vi "IT6700H Output DC Volts.vi"() -> ()   [LabVIEW 2015]
doc: "This example shows how to configure the instrument's output voltage level, over current protection, and over voltage protection. The actual voltage level and actual current level are returned as well as whether over voltage protection (OVP) or over current protection (OCP) has been tripped."
uses:
  <instrlib>/IT6700H/IT6700H.lvlib
panel:
  in  "OCP Level(A)":dbl min=0.0 format="%.2g"
  in  "OCP State":bool
  in  "OVP Level(V)":dbl min=0.0 format="%.2g"
  in  "OVP State":bool
  in  "Serial Configuration":T1={"Baud Rate"=9600, "Parity"=0, "Data Bits"=8, "Stop Bits"=10, "Flow Control"=0} {"Flow Control" items=["None", "XON/XOFF", "RTS/CTS", "XON/XOFF & RTS/CTS", "DTR/DSR", "XON/XOFF & DTR/DSR"]; "Stop Bits" items=["1.0"=10, "1.5"=15, "2.0"=20]; "Data Bits" items=["7"=7, "8"=8]; "Parity" items=["None", "Odd", "Even", "Mark", "Space"]; "Baud Rate" items=["300"=300, "600"=600, "1200"=1200, "2400"=2400, "4800"=4800, "9600"=9600, "19200"=19200]}
  in  "Stop Output":bool
  in  "Voltage(V)":dbl=1.0 min=0.0 format="%.2f"
  out "Read Current(A)":dbl format="%.3f"
  out "Read Voltage(V)":dbl format="%.3f"
  in  "Current(A)":dbl=1.0 min=0.0 format="%.2f"
  in  "VISA resource name":refnum<visa-resource-name>
  # "Source Output"
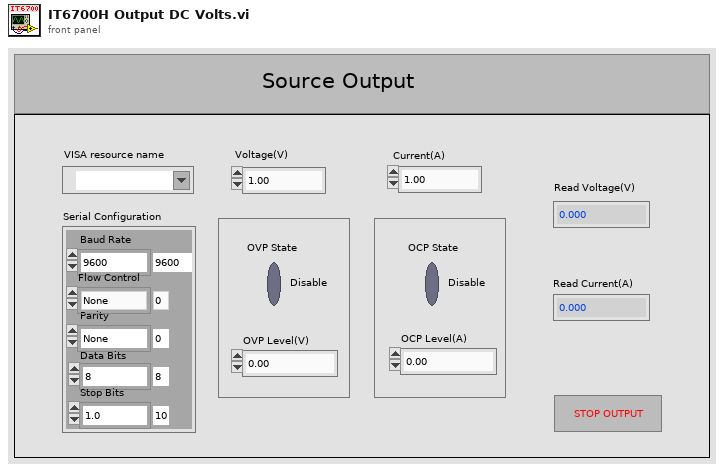
[diagram p1: front panel]
types:
  T1 = cluster{"Baud Rate":u32, "Parity":u16, "Data Bits":u16, "Stop Bits":u16, "Flow Control":u16}
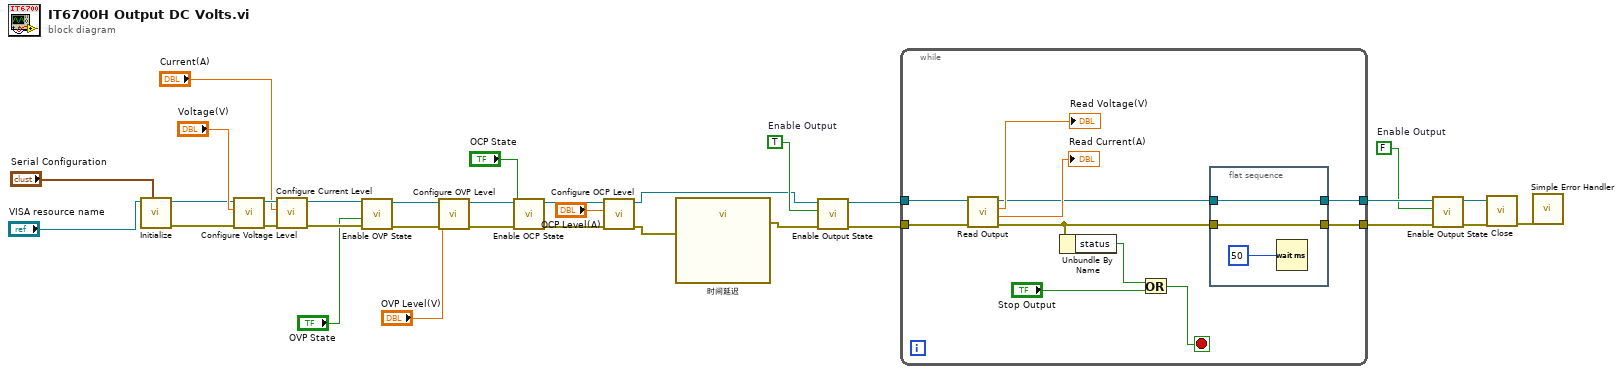
[diagram p0: block diagram]
diagram:
  w18 = FALSE  # Enable Output
  w23 = TRUE  # Enable Output
  n1 = call <instrlib>:"Initialize.vi"("Serial Configuration"="Serial Configuration", "VISA resource name"="VISA resource name") -> ("error out"=w16:errorcluster, "VISA resource name out"=w17:refnum<visa-resource-name>)  [unwired: 8 in]
  n2 = call <instrlib>:"Configure Voltage Level.vi"("error in"=w16, "Voltage(V)"="Voltage(V)", "VISA resource name"=w17) -> ("error out"=w29:errorcluster, "VISA resource name out"=w28:refnum<visa-resource-name>)  [unwired: 7 in]
  n3 = call <instrlib>:"Configure Current Level.vi"("error in"=w29, "Current(A)"="Current(A)", "VISA resource name"=w28) -> ("error out"=w14:errorcluster, "VISA resource name out"=w15:refnum<visa-resource-name>)  [unwired: 7 in]
  n4 = call <instrlib>:"Enable OVP State.vi"("error in"=w14, "State"="OVP State", "VISA resource name"=w15) -> ("error out"=w11:errorcluster, "VISA resource name out"=w12:refnum<visa-resource-name>)  [unwired: 7 in]
  n5 = call <instrlib>:"Configure OVP Level.vi"("error in"=w11, "Level(V)"="OVP Level(V)", "VISA resource name"=w12) -> ("error out"=w8:errorcluster, "VISA resource name out"=w9:refnum<visa-resource-name>)  [unwired: 7 in]
  n6 = call <instrlib>:"Enable OCP State.vi"("error in"=w8, "State"="OCP State", "VISA resource name"=w9) -> ("error out"=w5:errorcluster, "VISA resource name out"=w6:refnum<visa-resource-name>)  [unwired: 7 in]
  n7 = call <instrlib>:"Configure OCP Level.vi"("error in"=w5, "Level(A)"="OCP Level(A)", "VISA resource name"=w6) -> ("error out"=w2:errorcluster, "VISA resource name out"=w3:refnum<visa-resource-name>)  [unwired: 7 in]
  n8 = call "时间延迟"("error in (no error)"=w2) -> ("error out"=w1:errorcluster)  [unwired: 10 in]
  n9 = call <instrlib>:"Enable Output State.vi"("VISA resource name"=w3, "State"=w23, "error in"=w1) -> ("VISA resource name out"=w25:refnum<visa-resource-name>, "error out"=w24:errorcluster)  [unwired: 6 in]
  n10 = while {
    tunnel: w25 -> [w43]
    tunnel: w24 -> [w42]
    tunnel: [w36] -> w22
    tunnel: [w33] -> w21
    stop <- w37 stop-if-true
    n11 = call <instrlib>:"Read Output.vi"("error in"=w42, "VISA resource name"=w43) -> ("error out"=w34:errorcluster, "Actual Current Level (A)"=→"Read Current(A)":dbl, "Actual Voltage Level (V)"=→"Read Voltage(V)":dbl, "VISA resource name out"=w35:refnum<visa-resource-name>)  [unwired: 6 in]
    n12 = Unbundle By Name(w34) -> ("status"=w39:bool)
    n13 = Or(x=w39, y="Stop Output") -> (x .or. y?=w37:bool)
    n14 = flat-sequence {
      tunnel: [w46] -> w36
      tunnel: w35 -> [w46]
      tunnel: [w45] -> w33
      tunnel: w34 -> [w45]
      frame #0 {
        n15 = Wait (ms)(milliseconds to wait=50) -> ()  [unwired: 1 out]
      }
    }
  }
  n16 = call <instrlib>:"Enable Output State.vi"("VISA resource name"=w22, "State"=w18, "error in"=w21) -> ("VISA resource name out"=w20:refnum<visa-resource-name>, "error out"=w19:errorcluster)  [unwired: 6 in]
  n17 = call <instrlib>:"Close.vi"("error in"=w19, "VISA resource name"=w20) -> ("error out"=w26:errorcluster)  [unwired: 9 in]
  n18 = call <vilib>:"Simple Error Handler.vi"("error in (no error)"=w26) -> ()  [unwired: 4 in, 5 out]
